vi "Close Configuration Resource.vi"(8 "error in (no error)":errorcluster, 11 "database-configuration in":refnum<class "configuration-database.lvclass">) -> (0 "error out":errorcluster, 3 "database-configuration out":refnum<class "configuration-database.lvclass">)   [LabVIEW 2020, in "configuration-database.lvlib" / "configuration-database.lvclass"]
uses:
  configuration-database.lvclass
  externals/database-interface/IDatabase/IDatabase/IDatabase.lvclass
  IConfigDBQueries/IConfigurationDatabaseQueries.lvclass
  configuration-database.lvclass/configuration-database.ctl
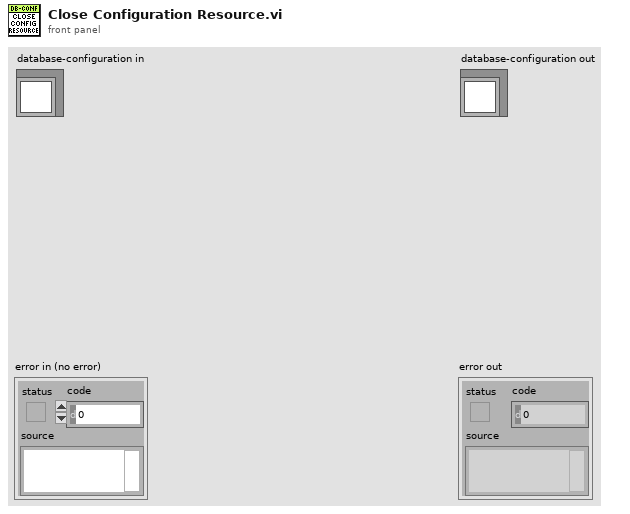
[diagram p1: front panel]
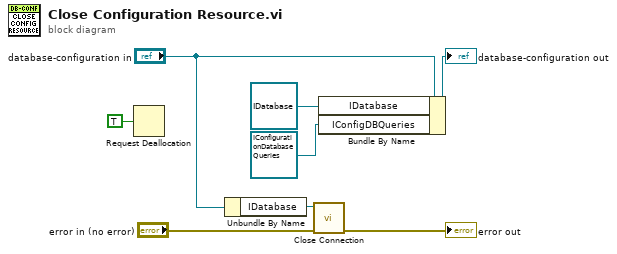
[diagram p0: block diagram]
diagram:
  n1 = Request Deallocation(TRUE ("flag")) -> ()
  n2 = Unbundle By Name("database-configuration in") -> ("IDatabase"=w7:refnum<class "IDatabase.lvclass">)
  n3 = call-dynamic "Close Connection.vi"("error in (no error)"="error in (no error)", "IDatabase in"=w7) -> ("error out"=→"error out":errorcluster)  [unwired: 8 in, 1 out]
  n4 = Bundle By Name(cluster="database-configuration in", "IDatabase"=refnum<class "IDatabase.lvclass"> refnum, "IConfigDBQueries"=refnum<class "IConfigurationDatabaseQueries.lvclass"> refnum) -> (→"database-configuration out":refnum<class "configuration-database.lvclass">)
